vi "Read Measurements.vi"(8 "error in (no error)":errorcluster, 11 "Compound Measurement in":refnum<class "Compound Measurement.lvclass">) -> (0 "error out":errorcluster, 2 "Measurements":string[](array[string]), 3 "Compound Measurement out":refnum<class "Compound Measurement.lvclass">)   [LabVIEW 2015, in "Compound Measurement.lvclass"]
uses:
  Compound Measurement.lvclass
  Compound Measurement.lvclass/Compound Measurement.ctl
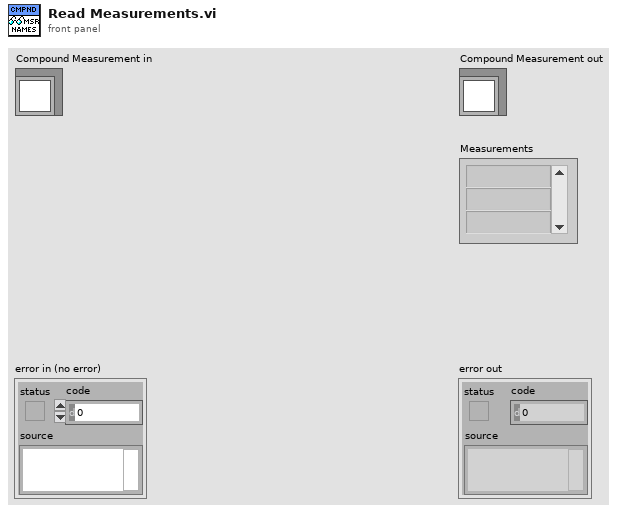
[diagram p1: front panel]
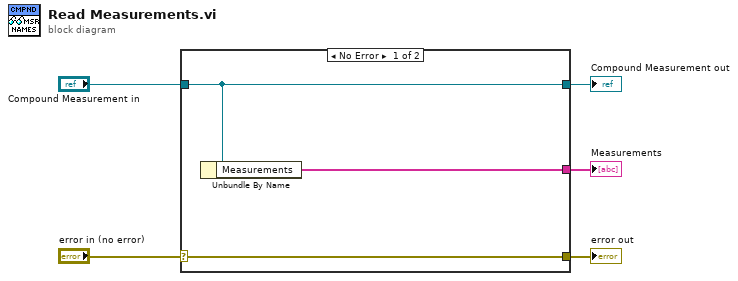
[diagram p0: block diagram]
diagram:
  n1 = case shown="No Error" "error in (no error)" {
    selector: "error in (no error)" -> [w8 w9]
    tunnel: [w8 w9] -> w4
    tunnel: [w7 w10] -> w2
    tunnel: "Compound Measurement in" -> [w7 w10]
    tunnel: [w6 _] -> w1
    frame No Error {
      n2 = Unbundle By Name(w7) -> ("Measurements"=w6:string[])
    }
    frame Error {
    }
  }
  "error out" <- w4
  "Compound Measurement out" <- w2
  "Measurements" <- w1
